vi "ArrayLoop.vi"() -> ()   [LabVIEW 2023]
uses:
  <vilib>/Analysis/NI_AALBase.lvlib
  <vilib>/Analysis/baseanly.llb/Mean (DBL).vi
panel:
  out "Numeric":i32
  in  "Array - Numeric":i32[](array[numeric])
  out "Array":i32[](array[numeric])
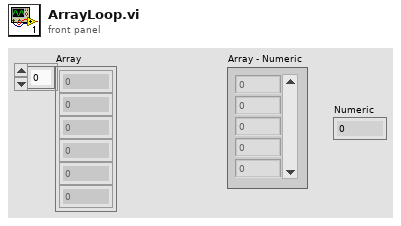
[diagram p1: front panel]
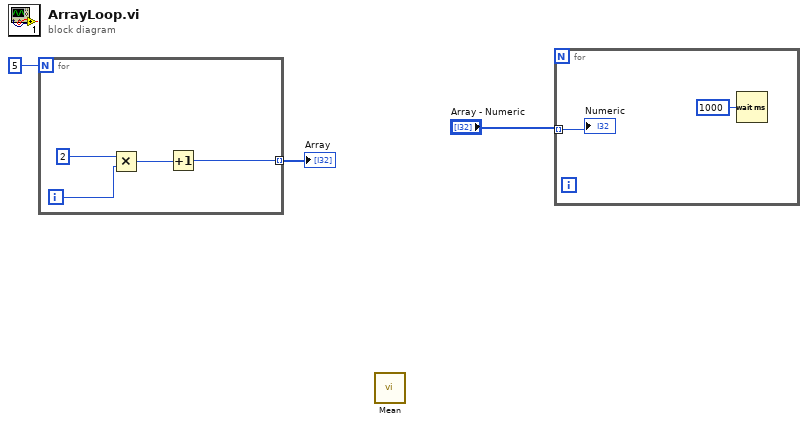
[diagram p0: block diagram]
diagram:
  n1 = for {
    N: 5 -> [_]
    tunnel: [w4] -> w2 mode=indexing
    i -> [w7]
    n2 = Multiply(x=2, y=w7) -> (x*y=w5:i32)
    n3 = Increment(x=w5) -> (x+1=w4:i32)
  }
  "Array" <- w2
  n4 = call-poly <vilib>:"Mean.vi"() -> ()  [unwired: 1 in, 2 out]
  n5 = for {
    tunnel: "Array - Numeric" -> [w9] mode=indexing
    n6 = Wait (ms)(milliseconds to wait=u32 1000) -> ()  [unwired: 1 out]
    "Numeric" <- w9
  }
